vi "DyMIN_UpdateFPGAFrontPanel.vi"(8 "error in (no error)":errorcluster, 11 "FPGA Interface":T1) -> (0 "error out":errorcluster, 3 "FPGA VI Reference Out":T1)   [LabVIEW 2016]
uses:
  DyMIN_FPGA_Main reference.ctl
  <vilib>/Utility/error.llb/Error Cluster From Error Code.vi
  <vilib>/rvi/errors/niLvFpgaAdjustHostInterfaceError.vi
  <vilib>/rvi/interface/nirviReadWriteControl/nirviReadWriteControl.xnode
  FPGA Bitfiles/Dymin4ALL_FPGATarget_DyminFPGAMain2_xawG5vdEA4w.lvbitx
  Dymin_FPGA_Main.vi
  NiFpgaLv.dll
panel:
  in  "Columns":u16=16
  in  "Rows":u16=16
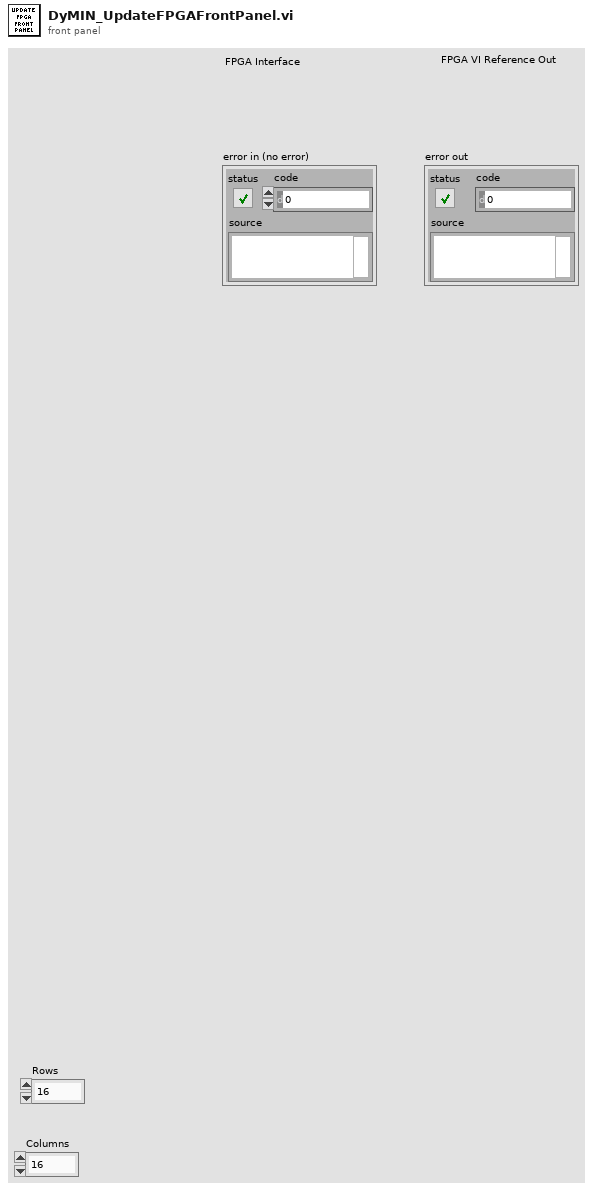
[diagram p1: front panel]
types:
  T1 = typedef "DyMIN_FPGA_Main reference.ctl" = refnum<k20>
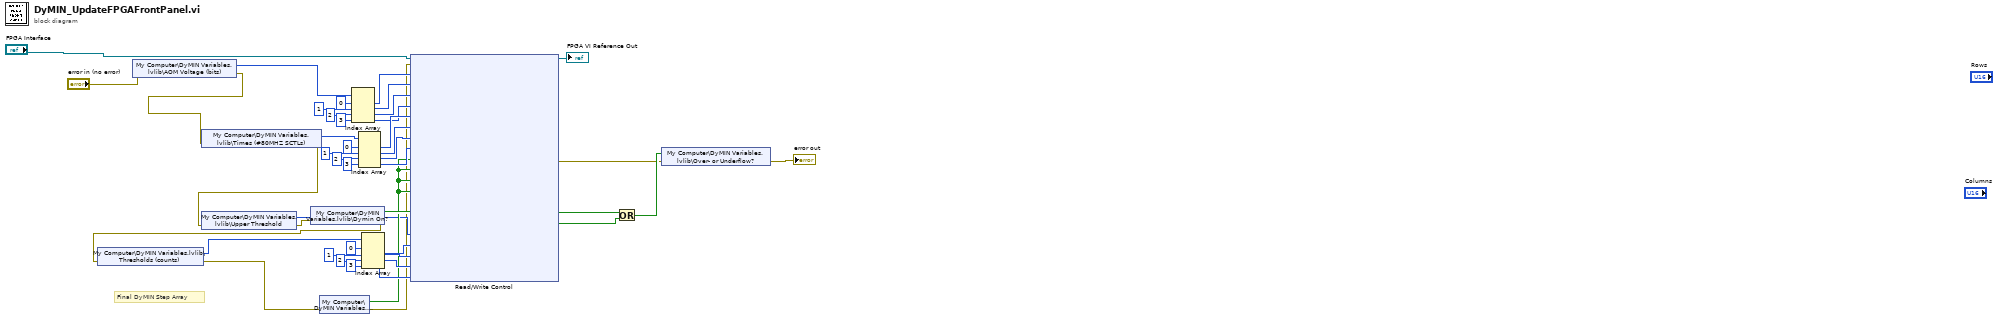
[diagram p0: block diagram]
diagram:
  # "Final DyMIN Step Array"
  n1 = shared-variable "My Computer\\DyMIN Variables.lvlib\\AOM Voltage (bits)"(error in="error in (no error)") -> (w17:u16[], error out=w1:errorcluster)
  n2 = shared-variable "My Computer\\DyMIN Variables.lvlib\\Times (#80MHZ SCTLs)"(error in=w1) -> (w16:u32[], error out=w11:errorcluster)
  n3 = shared-variable "My Computer\\DyMIN Variables.lvlib\\Upper Threshold"(error in=w11) -> (w14:u32, error out=w10:errorcluster)
  n4 = shared-variable "My Computer\\DyMIN Variables.lvlib\\Dymin On?"(error in=w10) -> (w18:bool, error out=w9:errorcluster)
  n5 = shared-variable "My Computer\\DyMIN Variables.lvlib\\Thresholds (counts)"(error in=w9) -> (w13:u32[], error out=w4:errorcluster)
  n6 = shared-variable "My Computer\\DyMIN Variables.lvlib\\Stop"(error in=w4) -> (w15:bool, error out=w8:errorcluster)
  n7 = Index Array(array=w17, index #1=0 ("index"), index #2=1 ("index"), index #3=2 ("index"), index #4=3 ("index")) -> (element #1=w25:u16, element #2=w26:u16, element #3=w27:u16, element #4=w28:u16)
  n8 = Index Array(array=w16, index #1=0 ("index"), index #2=1 ("index"), index #3=2 ("index"), index #4=3 ("index")) -> (element #1=w33:u32, element #2=w34:u32, element #3=w35:u32, element #4=w36:u32)
  n9 = Index Array(array=w13, index #1=0 ("index"), index #2=1 ("index"), index #3=2 ("index"), index #4=3 ("index")) -> (element #1=w41:u32, element #2=w42:u32, element #3=w43:u32, element #4=w44:u32)
  n10 = xnode ("Read/Write Control")("FPGA VI Reference In"="FPGA Interface", "error in"=w8, "V0"=w25, "V1"=w26, "V2"=w27, "V3"=w28, "t0"=w33, "t1"=w34, "t2"=w35, "t3"=w36, "stop 1"=w15, "stop 2"=w15, "stop 3"=w15, "stop 4"=w15, "Dymin On?"=w18, "Upper Threhold (counts)"=w14, "T0"=w41, "T1"=w42, "T2"=w43, "T3"=w44) -> ("FPGA VI Reference Out"=→"FPGA VI Reference Out":T1, "error out"=w7:errorcluster, "Overflow1"=w19:bool, "Overflow2"=w20:bool)
  n11 = Or(x=w19, y=w20) -> (x .or. y?=w12:bool)
  n12 = shared-variable "My Computer\\DyMIN Variables.lvlib\\Over- or Underflow?"(w12, error in=w7) -> (error out=→"error out":errorcluster)
